vi "Go to temperature and wait until there.vi"(7 "Wait time before change":dbl[unit], 8 "error in (no error)":errorcluster, 9 "Wait time after change":dbl[unit]=720.0, 10 "Go to temperture":dbl, 11 "VISA resource name":refnum<visa-resource-name>="COM3") -> (0 "error out":errorcluster, 3 "VISA resource name out":refnum<visa-resource-name>)   [LabVIEW 2017]
doc: "This changes the temperature setpoint. If you want to query the setpoint after this, make sure there is a 0.2 s delay (according to manual)."
panel:
  out "Current actual temperature":dbl
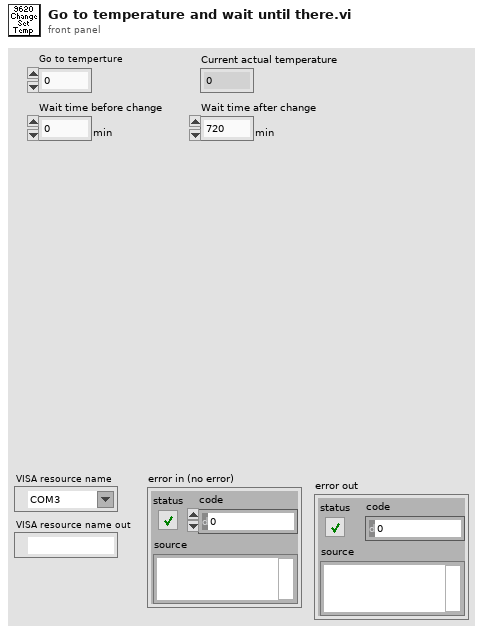
[diagram p1: front panel]
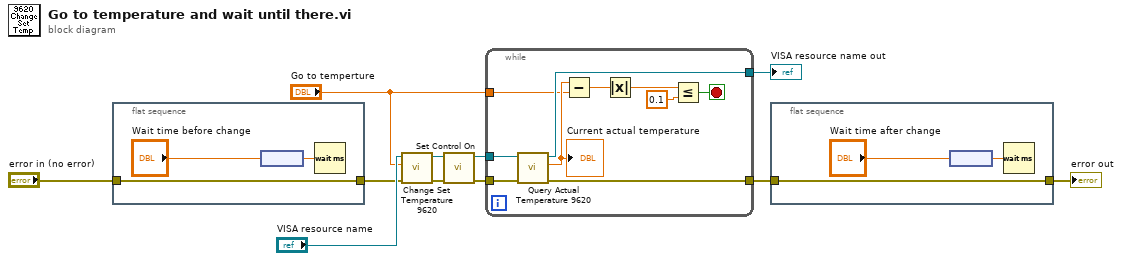
[diagram p0: block diagram]
diagram:
  n1 = flat-sequence {
    tunnel: [w12] -> w1
    tunnel: "error in (no error)" -> [w12]
    frame #0 {
      n2 = node("Wait time before change") -> (w13:dbl)
      n3 = Wait (ms)(milliseconds to wait=w13) -> ()  [unwired: 1 out]
    }
  }
  n4 = call "Change Set Temperature 9620.vi"("error in (no error)"=w1, "Temperture Setpoint"="Go to temperture", "VISA resource name"="VISA resource name") -> ("error out"=w6:errorcluster, "VISA resource name out"=w8:refnum<visa-resource-name>)  [unwired: 7 in]
  n5 = call "Set Control On.vi"("error in (no error)"=w6, "VISA resource name"=w8) -> ("error out"=w5:errorcluster, "VISA resource name out"=w7:refnum<visa-resource-name>)  [unwired: 8 in]
  n6 = while {
    tunnel: w5 -> [w24]
    tunnel: [w23] -> w4
    tunnel: w7 -> [w22]
    tunnel: [w21] -> w10
    tunnel: "Go to temperture" -> [w19]
    stop <- w15 stop-if-true
    n7 = call "Query Actual Temperature 9620.vi"("error in (no error)"=w24, "VISA resource name"=w22) -> ("error out"=w23:errorcluster, "Current actual temperature"=w20:dbl, "VISA resource name out"=w21:refnum<visa-resource-name>)  [unwired: 7 in]
    "Current actual temperature" <- w20
    n8 = Subtract(x=w20, y=w19) -> (x-y=w18:dbl)
    n9 = Absolute Value(x=w18) -> (abs(x)=w17:dbl)
    n10 = Less Or Equal?(x=w17, y=0.1) -> (x <= y?=w15:bool)
  }
  "VISA resource name out" <- w10
  n11 = flat-sequence {
    tunnel: [w27] -> w3
    tunnel: w4 -> [w27]
    frame #0 {
      n12 = node("Wait time after change") -> (w25:dbl)
      n13 = Wait (ms)(milliseconds to wait=w25) -> ()  [unwired: 1 out]
    }
  }
  "error out" <- w3
